vi "NewtonsPSM_Meas_Harm.vi"(0 "VISA session":refnum<visa-resource-name>, 11 "error in (no error)":errorcluster) -> (4 "dup VISA session":refnum<visa-resource-name>, 6 "Read Strings":string, 8 "Measure":dbl[](array[numeric]) format="%^.4e", 15 "error out":errorcluster)   [LabVIEW 2025, in "NewtonsPSM1735.lvlib"]
doc: "This VI reads the Harmonic Measurement from the PPA2530"
uses:
  NewtonsPSM1735.lvlib
panel:
  # "Freq"
  # "Mag Ch2"
  # "Harm Ch1"
  # "Harm Ch2"
  # "Harm Ch2(%)"
  # "Harm Ch1(%)"
  # "Mag Ch1"
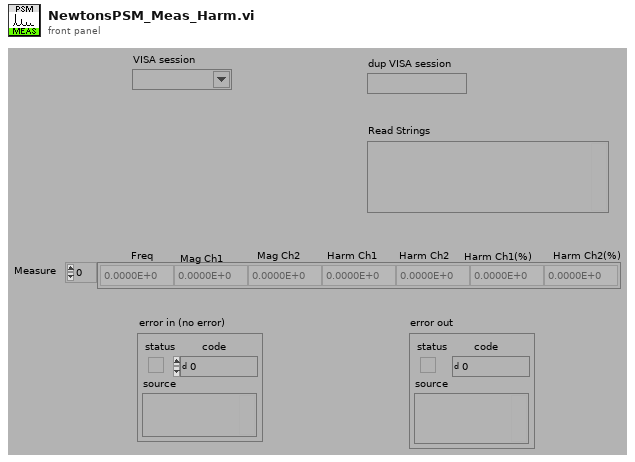
[diagram p1: front panel]
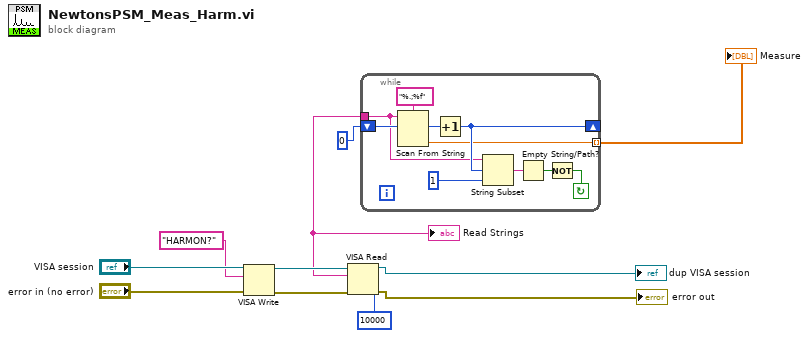
[diagram p0: block diagram]
diagram:
  n1 = VISA Write(VISA resource name="VISA session", write buffer="HARMON?", error in (no error)="error in (no error)") -> (VISA resource name out=w8:refnum<visa-resource-name>, error out=w7:errorcluster)  [unwired: 1 out]
  n2 = VISA Read(VISA resource name=w8, byte count=u32 10000 ("ÊÞ²Ä¶³ÝÄi0j"), error in (no error)=w7) -> (VISA resource name out=→"dup VISA session":refnum<visa-resource-name>, read buffer=w4:string, error out=→"error out":errorcluster)  [unwired: 1 out]
  "Read Strings" <- w4
  n3 = while {
    tunnel: [w14] -> w5 mode=indexing
    shift-left: 0 -> [w13]
    shift-right: [w17] -> _
    tunnel: w4 -> [w12]
    stop <- w18 continue-if-true
    n4 = Scan From String(format string="%.;%f", input string=w12, initial scan location=w13) -> (offset past scan=w15:u32, output 1=w14:dbl)  [unwired: 1 in, 3 out]
    n5 = Increment(x=w15) -> (x+1=w17:u32)
    n6 = String Subset(string=w12, offset (0)=w17, length (rest)=1) -> (substring=w20:string)
    n7 = Empty String/Path?(string/path=w20) -> (empty?=w19:bool)
    n8 = Not(x=w19) -> (.not. x?=w18:bool)
  }
  "Measure" <- w5
